vi "Translate Lidar Coords to Grid.vi"(11 "Obstacle Avoidance Data":T1) -> (3 "Obstacle Avoidance Data":T1)   [LabVIEW 2017]
uses:
  <vilib>/Analysis/coordinate.llb/2D Cartesian Coordinate Shift (Scalar).vi
  <vilib>/Analysis/NI_AALPro.lvlib
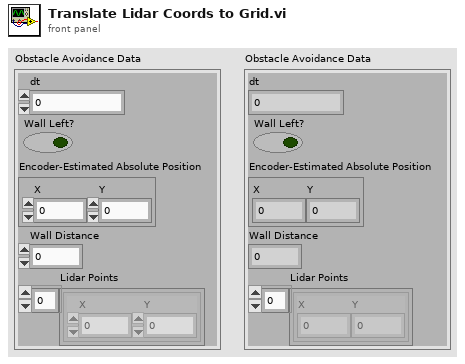
[diagram p1: front panel]
types:
  T1 = cluster{"dt":dbl, "Wall Left?":bool, "Encoder-Estimated Absolute Position":cluster{"X":dbl, "Y":dbl}, "Wall Distance":dbl, "Lidar Points":cluster{"X":dbl, "Y":dbl}[]}
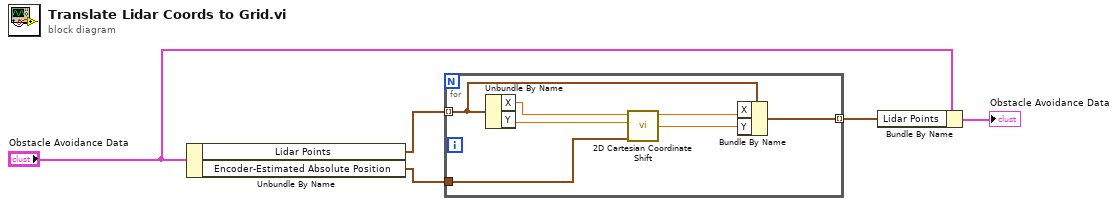
[diagram p0: block diagram]
diagram:
  n1 = Unbundle By Name("Obstacle Avoidance Data") -> ("Lidar Points"=w5:cluster{"X":dbl, "Y":dbl}[], "Encoder-Estimated Absolute Position"=w4:cluster{"X":dbl, "Y":dbl})
  n2 = for {
    tunnel: w5 -> [w12] mode=indexing
    tunnel: [w11] -> w3 mode=indexing
    tunnel: w4 -> [w6]
    n3 = Unbundle By Name(w12) -> ("X"=w8:dbl, "Y"=w7:dbl)
    n4 = call-poly <vilib>:"2D Cartesian Coordinate Shift.vi"("shift"=w6, "y"=w7, "x"=w8) -> ("y out"=w9:dbl, "x out"=w10:dbl)  [unwired: 6 in, 1 out]
    n5 = Bundle By Name(cluster=w12, "X"=w10, "Y"=w9) -> (w11:cluster{"X":dbl, "Y":dbl})
  }
  n6 = Bundle By Name(cluster="Obstacle Avoidance Data", "Lidar Points"=w3) -> (→"Obstacle Avoidance Data":T1)
